vi "TCPHandler.vi"(0 "connection ID":refnum<k5>, 5 "results_cluster":refnum<vi>[](array[refnum]), 7 "params_cluster":refnum<vi>[](array[refnum]), 9 "method":string, 11 "error":errorcluster) -> (4 "connection ID":refnum<k5>, 6 "JSON-request":string, 8 "JSON-response":string="{\"jsonrpc\":\"2.0\",\"method\":\"\",\"params\":[5,1.245,true,\"name\"],\"id\":\"1\"}", 15 "error":errorcluster)   [LabVIEW 2016, in "AMC_VIs.lvlib"]
uses:
  AMC_VIs.lvlib
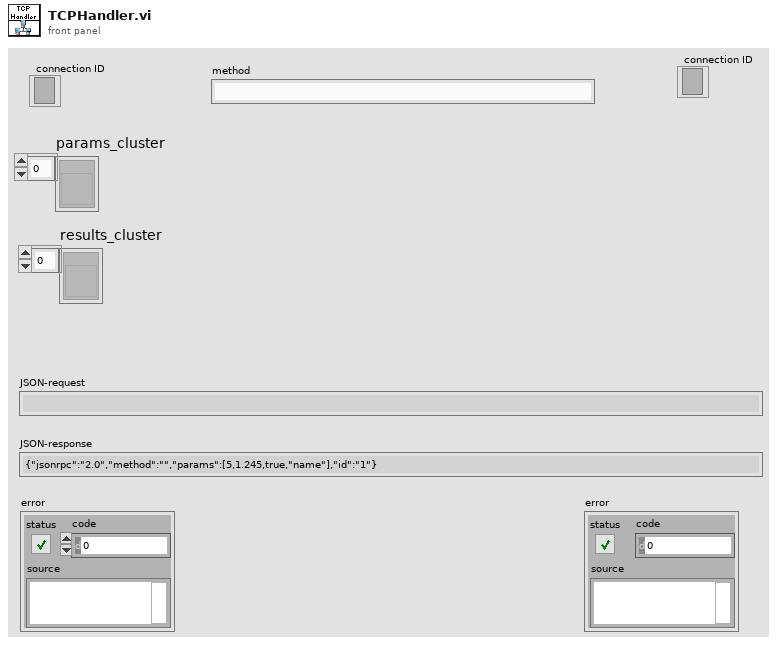
[diagram p1: front panel]
types:
  T1 = enum16{"Standard", "Buffered", "CRLF", "Immediate"}
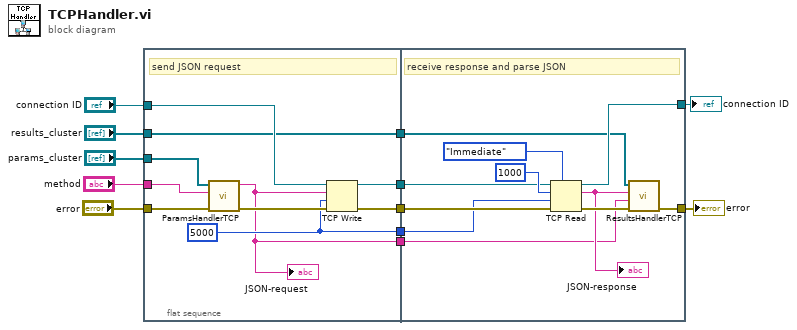
[diagram p0: block diagram]
diagram:
  n1 = flat-sequence {
    tunnel: "connection ID" -> [w22]
    tunnel: "method" -> [w19]
    tunnel: [w20] -> w9
    tunnel: [w21] -> w8
    tunnel: "error" -> [w18]
    tunnel: "params_cluster" -> [w17]
    tunnel: [w15] -> w4
    tunnel: "results_cluster" -> [w14]
    tunnel: [w14] -> w2
    tunnel: [w13] -> w1
    tunnel: [w29] -> w11
    tunnel: w9 -> [w31]
    tunnel: w8 -> [w30]
    tunnel: [w28] -> w6
    tunnel: w4 -> [w27]
    tunnel: w2 -> [w26]
    tunnel: w1 -> [w23]
    frame #0 {
      w15 = 5000 ("timeout ms (25000)")
      # "send JSON request"
      n2 = call "ParamsHandlerTCP.vi"("error"=w18, "method"=w19, "params_cluster"=w17) -> ("error"=w16:errorcluster, "JSON-request"=w13:string)  [unwired: 6 in]
      "JSON-request" <- w13
      n3 = TCP Write(connection ID=w22, data in=w13, error in (no error)=w16, 9:w15) -> (connection ID out=w20:refnum<k5>, error out=w21:errorcluster)  [unwired: 1 out]
    }
    frame #1 {
      # "receive response and parse JSON"
      n4 = TCP Read(connection ID=w31, bytes to read=1000, error in (no error)=w30, 7:T1."Immediate" ("mode (standard)"), 9:w27) -> (connection ID out=w29:refnum<k5>, data out=w24:string, error out=w25:errorcluster)
      "JSON-response" <- w24
      n5 = call "ResultsHandlerTCP.vi"("error"=w25, "JSON-request"=w23, "JSON-response"=w24, "results_cluster"=w26) -> ("error"=w28:errorcluster)  [unwired: 7 in]
    }
  }
  "connection ID" <- w11
  "error" <- w6
